vi "Handle Command.vi"(8 "error in (no error)":errorcluster, 9 "Data":variant, 10 "Command":string, 11 "Example Instrument in":refnum<class "Example Instrument.lvclass">) -> (0 "error out":errorcluster, 1 "Processed Data":variant, 2 "Command":string, 3 "Example Instrument out":refnum<class "Example Instrument.lvclass">)   [LabVIEW 2016, in "Example Instrument.lvclass"]
uses:
  Example Instrument.lvclass
  Typedefs/getAll--Cluster.ctl
  Instrument/Instrument.lvclass
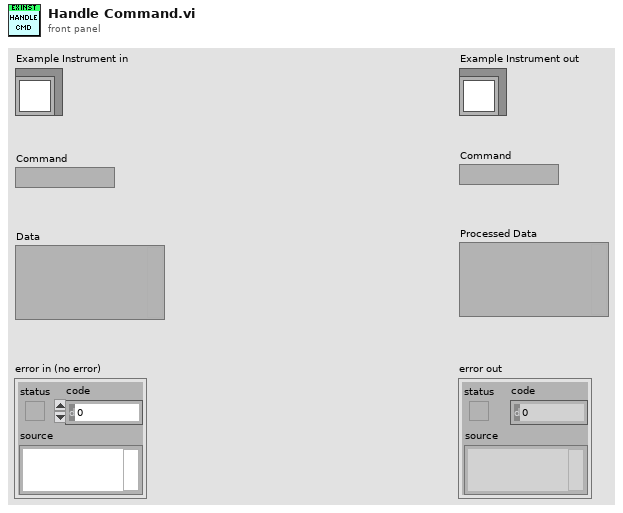
[diagram p1: front panel]
types:
  T1 = typedef "Example Instrument.lvclass/getAll--Cluster.ctl" = cluster{"Levy 1":dbl, "Logger SMO":dbl, "SMO Boolean":bool, "SMO String":string}
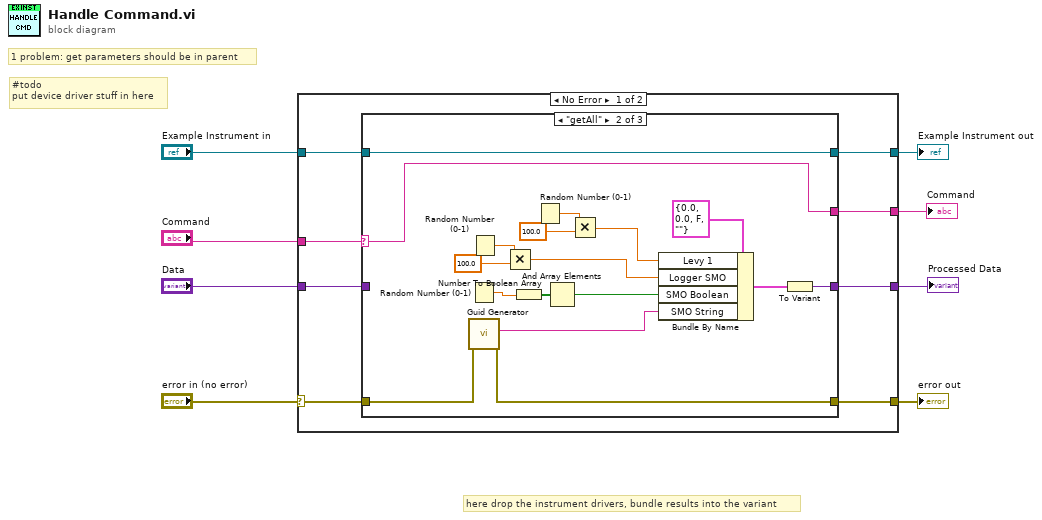
[diagram p0: block diagram]
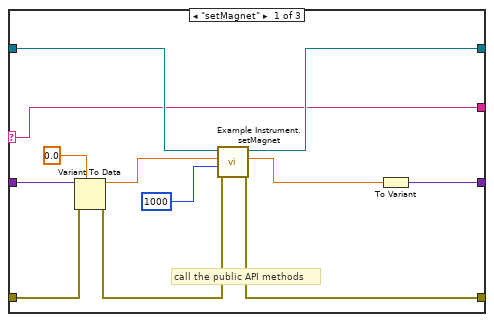
[diagram p2: hidden frame]
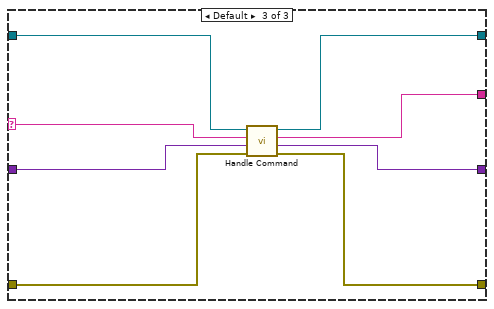
[diagram p3: hidden frame]
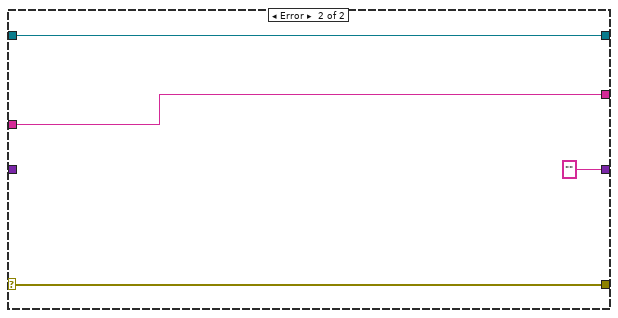
[diagram p4: hidden frame]
diagram:
  # "here drop the instrument drivers, bundle results into the variant"
  # "1 problem: get parameters should be in parent"
  # "#todo\nput device driver stuff in here"
  n1 = case shown="No Error" "error in (no error)" {
    selector: "error in (no error)" -> [w12 w57]
    tunnel: [w10 w57] -> w6
    tunnel: [w14 w56] -> w5
    tunnel: "Example Instrument in" -> [w15 w56]
    tunnel: "Command" -> [w16 w54]
    tunnel: [w13 "" ("String")] -> w3
    tunnel: "Data" -> [w11 _]
    tunnel: [w9 w54] -> w1
    frame No Error {
      n2 = case shown="\"getAll\"" w16 {
        selector: w16 -> [w17 w32 w53]
        tunnel: w15 -> [w28 w45 w50]
        tunnel: [w27 w45 w47] -> w14
        tunnel: [w18 w33 w49] -> w13
        tunnel: w12 -> [w21 w30 w51]
        tunnel: w11 -> [w26 _ w52]
        tunnel: [w23 w31 w48] -> w10
        tunnel: [w17 w32 w46] -> w9
        frame "setMagnet" {
          # "call the public API methods"
          n3 = Variant To Data(error in=w21, type=0.0, Variant=w26) -> (data=w25:dbl, error out=w22:errorcluster)
          n4 = call "Example Instrument.setMagnet.vi"("error in (no error)"=w22, "timeout in ms (1000)"=1000, "setMagnet"=w25, "Example Instrument"=w28) -> ("error out"=w23:errorcluster, "notification"=w19:dbl, "Example Instrument out"=w27:refnum<class "Example Instrument.lvclass">)  [unwired: 4 in, 1 out]
          n5 = To Variant(anything=w19) -> (Variant=w18:variant)
        }
        frame "getAll" {
          n6 = Random Number (0-1)() -> (number: 0 to 1=w40:dbl)
          n7 = call <vilib>:"Guid Generator.vi"("error in (no error)"=w30) -> ("error out"=w31:errorcluster, "GUID"=w29:string)  [unwired: 9 in]
          n8 = Random Number (0-1)() -> (number: 0 to 1=w42:dbl)
          n9 = Multiply(x=w42, y=100.0) -> (x*y=w37:dbl)
          n10 = Number To Boolean Array(number=w40) -> (Boolean array=w39:bool[])
          n11 = Random Number (0-1)() -> (number: 0 to 1=w43:dbl)
          n12 = And Array Elements(Boolean array=w39) -> (logical AND=w36:bool)
          n13 = Multiply(x=w43, y=100.0) -> (x*y=w38:dbl)
          n14 = Bundle By Name(cluster=T1 {"Levy 1"=0.0, "Logger SMO"=0.0, "SMO Boolean"=FALSE, "SMO String"=""}, "Levy 1"=w38, "Logger SMO"=w37, "SMO Boolean"=w36, "SMO String"=w29) -> (w35:T1)
          n15 = To Variant(anything=w35) -> (Variant=w33:variant)
        }
        frame Default {
          n16 = call-parent "Handle Command.vi"("error in (no error)"=w51, "Data"=w52, "Command"=w53, "Instrument in"=w50) -> ("error out"=w48:errorcluster, "Processed Data"=w49:variant, "Command"=w46:string, "Instrument out"=w47:refnum<class "Example Instrument.lvclass">)  [unwired: 4 in]
        }
      }
    }
    frame Error {
    }
  }
  "error out" <- w6
  "Example Instrument out" <- w5
  "Command" <- w1
  "Processed Data" <- w3
